vi "Read PS Driver.vi"(8 "error in (no error)":errorcluster, 11 "PS Control Persistence Actor in":refnum<class "PS Control Persistence Actor.lvclass">) -> (0 "error out":errorcluster, 2 "PS Driver.lvlib:PS Driver.lvclass":refnum<class "PS Driver.lvclass">, 3 "PS Control Persistence Actor out":refnum<class "PS Control Persistence Actor.lvclass">)   [LabVIEW 2025, in "PS Control Persistence.lvlib" / "PS Control Persistence Actor.lvclass"]
doc: "Author: Scott Hannahs <sth@magnet.fsu.edu>\n\nThis software is licensed for use under the “MIT License\"\nCopyright (c) 2025 Scott Hannahs, sth@sth@magnet.sthnet.net\n\nPermission is hereby granted, free of charge, to any person obtaining a copy of this software and associated documentation files (the \"Software\"), to deal in the Software without restriction, including without limitation the rights to use, copy, modify, merge, publish, distribute, sublicense, and/or sell copies of the Software, and to permit persons to whom the Software is furnished to do so, subject to the following conditions: The above copyright notice and this permission notice shall be included in all copies or substantial portions of the Software.\n\nTHE SOFTWARE IS PROVIDED \"AS IS\", WITHOUT WARRANTY OF ANY KIND, EXPRESS OR IMPLIED, INCLUDING BUT NOT LIMITED TO THE WARRANTIES OF MERCHANTABILITY, FITNESS FOR A PARTICULAR PURPOSE AND NONINFRINGEMENT. IN NO EVENT SHALL THE AUTHORS OR COPYRIGHT HOLDERS BE LIABLE FOR ANY CLAIM, DAMAGES OR OTHER LIABILITY, WHETHER IN AN ACTION OF CONTRACT, TORT OR OTHERWISE, ARISING FROM, OUT OF OR IN CONNECTION WITH THE SOFTWARE OR THE USE OR OTHER DEALINGS IN THE SOFTWARE."
uses:
  PS Control Persistence Actor.lvclass
  PS Driver/PS Driver.lvclass
  PS Control Persistence Actor.lvclass/PS Control Persistence Actor.ctl
  PS Driver/PS Driver with Persistence.lvclass
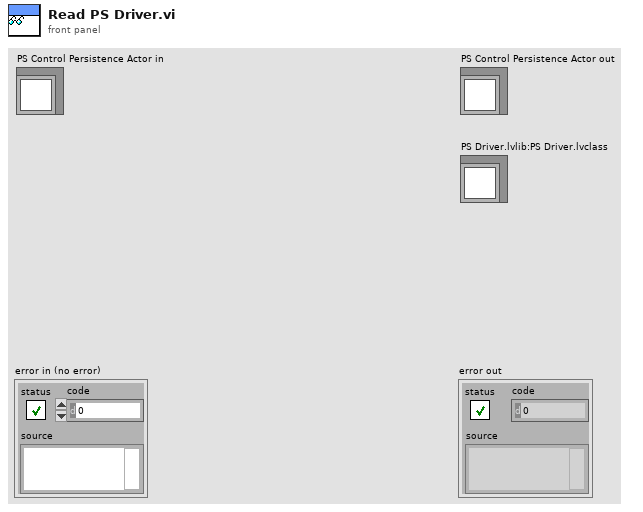
[diagram p1: front panel]
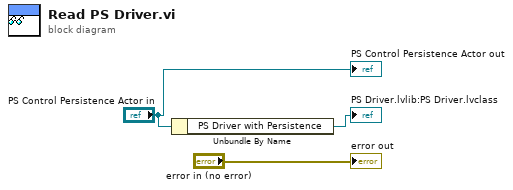
[diagram p0: block diagram]
diagram:
  n1 = Unbundle By Name("PS Control Persistence Actor in") -> ("PS Driver with Persistence"=→"PS Driver.lvlib:PS Driver.lvclass":refnum<class "PS Driver with Persistence.lvclass">)
  "error out" <- "error in (no error)"
  "PS Control Persistence Actor out" <- "PS Control Persistence Actor in"
